vi "Autonomous Independent.vi"   [LabVIEW 2019]
doc: "This VI is called when autonomous begins, and will automatically be terminated when autonomous ends. You can carry out timed or sensor driven robot movement independently without needing to return to the caller."
uses:
  <vilib>/Rock Robotics/WPI/Utilities/WPI_GetSetVariantRefNum.vi
  <vilib>/Rock Robotics/Network Tables/NT Read String.vi
  <vilib>/Rock Robotics/Network Tables/NT Write Numeric Array.vi
  Robot Global Data.vi
panel:
  # "Be sure to right-click and choose Data Operations>>Make Current Value default if you want to save the array values with the VI"
types:
  T1 = typedef "WPI_JoystickDevRef.ctl" = cluster{"Device":T2}
  T2 = typedef "WPI_JoystickDeviceEnum.ctl" = enum16{"USB 0", "USB 1", "USB 2", "USB 3", "USB 4", "USB 5"}
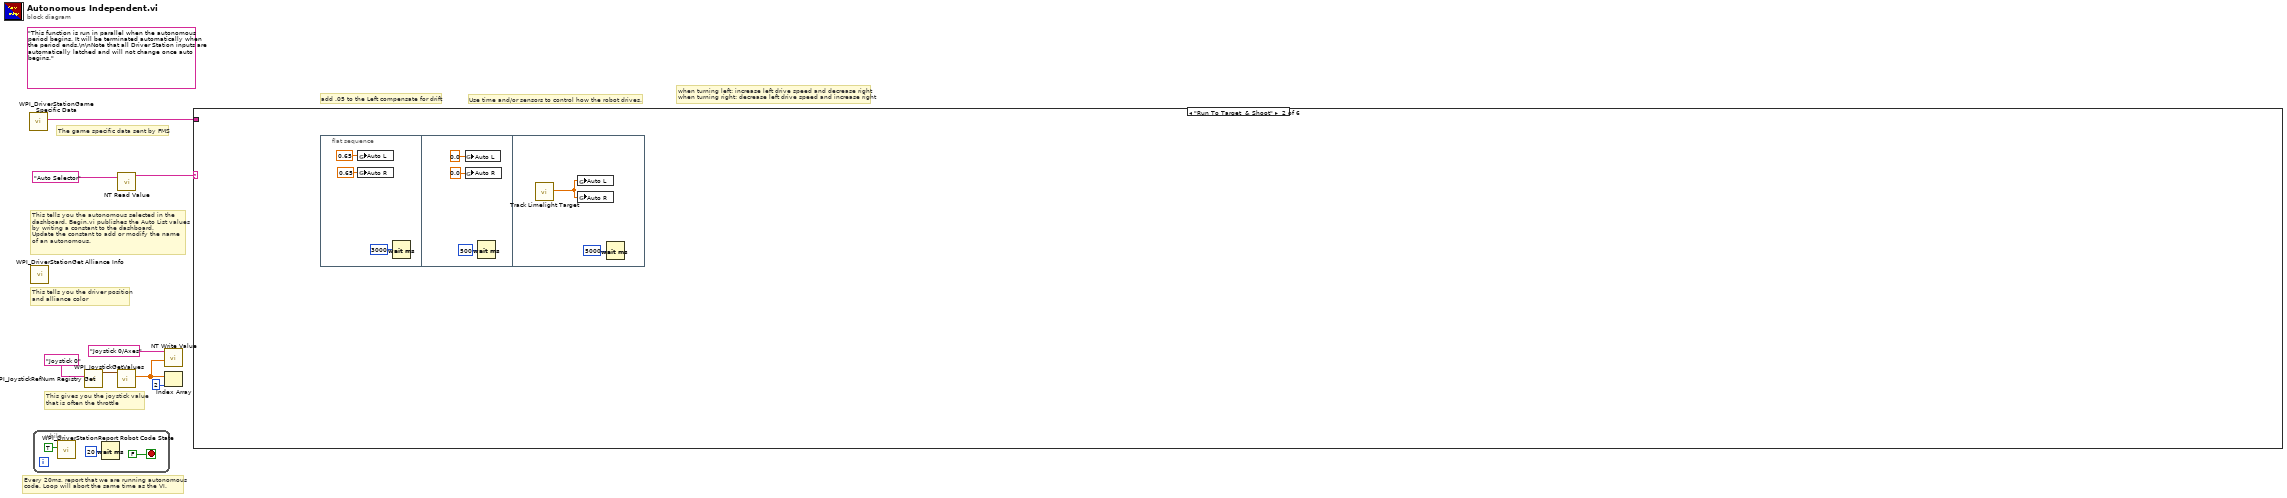
[diagram p0: block diagram]
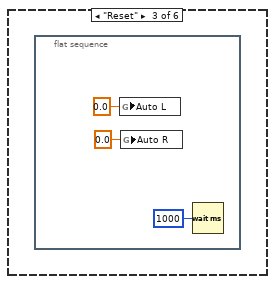
[diagram p3: hidden frame]
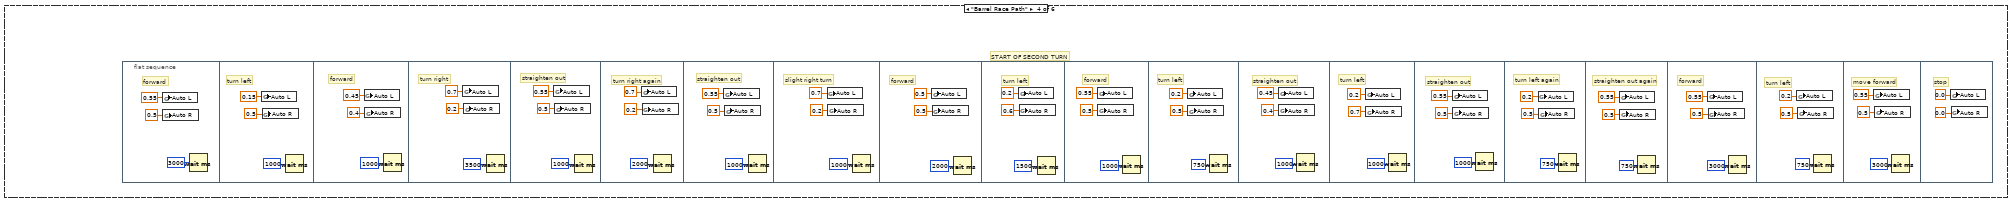
[diagram p4: hidden frame]
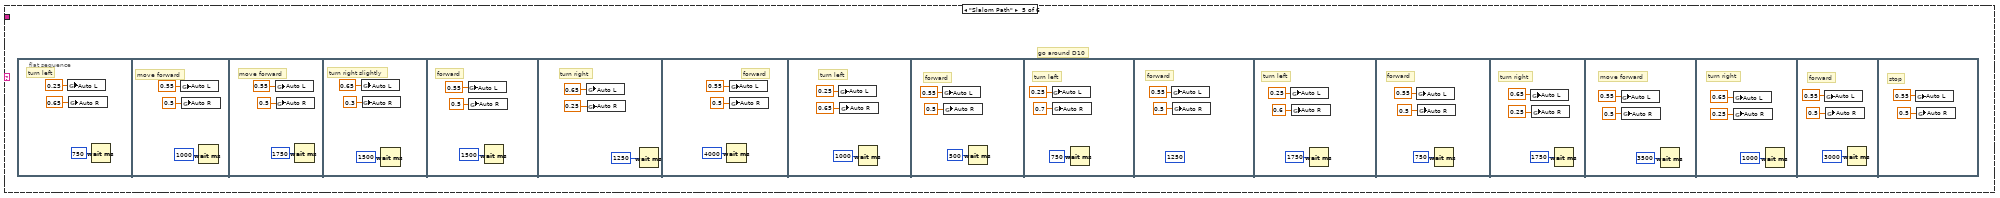
[diagram p5: hidden frame]
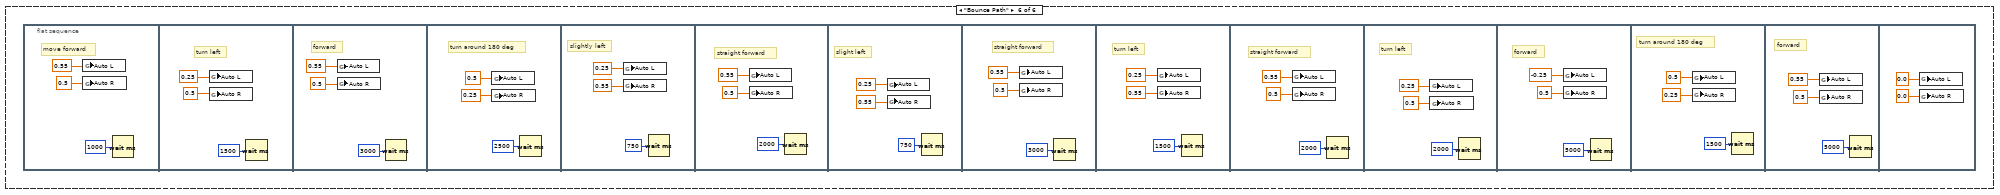
[diagram p6: hidden frame]
diagram:
  (unwired) "This function is run in parallel when the autonomous period begins. It will be terminated automatically when the period ends.\n\nNote that all Driver Station inputs are automatically latched and will not change once auto begins."
  # "add .05 to the Left compensate for drift"
  # "when turning left: increase left drive speed and decrease right\nwhen turning right: decrease left drive speed and increase right"
  # "The game specific data sent by FMS"
  # "This tells you the autonomous selected in the \ndashboard. Begin.vi publishes the Auto List values\nby writing a constant to the dashboard.\nUpdate the constant to add or modify the name\nof an autonomous."
  # "Every 20ms, report that we are running autonomous\ncode. Loop will abort the same time as the VI."
  # "This gives you the joystick value\nthat is often the throttle"
  # "Use time and/or sensors to control how the robot drives."
  # "This tells you the driver position\nand alliance color"
  n1 = call <vilib>:"WPI_DriverStationGame Specific Data.vi"() -> ("Game Specific Data"=w1:string)  [unwired: 11 in]
  n2 = call <vilib>:"WPI_DriverStationGet Alliance Info.vi"() -> ()  [unwired: 12 out]
  n3 = while {
    stop <- FALSE stop-if-true
    n4 = call <vilib>:"WPI_DriverStationReport Robot Code State.vi"("Autonomous"=TRUE) -> ()  [unwired: 10 in, 1 out]
    n5 = Wait (ms)(milliseconds to wait=u32 20) -> ()  [unwired: 1 out]
  }
  n6 = call <vilib>:"WPI_JoystickRefNum Registry Get.vi"("refnum name"="Joystick 0") -> ("JoystickDevRef"=w7:T1)  [unwired: 1 in, 9 out]
  n7 = call <vilib>:"WPI_JoystickGetValues.vi"("JoystickDevRef"=w7) -> ("Axes"=w3:dbl[])  [unwired: 6 in, 4 out]
  n8 = call-poly <vilib>:"NT Read Value.vi"("Name"="Auto Selector") -> ("String"=w4:string)  [unwired: 9 in, 1 out]
  n9 = call-poly <vilib>:"NT Write Value.vi"("Numeric Array"=w3, "Name"="Joystick 0/Axes") -> ()  [unwired: 9 in, 1 out]
  n10 = Index Array(array=w3, index=2) -> ()  [unwired: 1 out]
  n11 = case shown="\"Run To Target  & Shoot\"" w4 {
    tunnel: w1 -> [_ _ _ _ _ _]
    frame Default {
      # "You can put your main auto here, or you can right-click on the case and make any\nother frame be the default case."
      # "This is the frame that will execute if no selection is made, or if it is not recognized"
    }
    frame "Run To Target  & Shoot" {
      n12 = flat-sequence {
        frame #0 {
          n13 = global write "Robot Global Data.vi" "Auto L"(0.65 ("Auto L")) -> ()
          n14 = global write "Robot Global Data.vi" "Auto R"(0.65 ("Auto R")) -> ()
          n15 = Wait (ms)(milliseconds to wait=u32 3000) -> ()  [unwired: 1 out]
        }
        frame #1 {
          n16 = global write "Robot Global Data.vi" "Auto L"(0.0 ("Auto L")) -> ()
          n17 = global write "Robot Global Data.vi" "Auto R"(0.0 ("Auto R")) -> ()
          n18 = Wait (ms)(milliseconds to wait=u32 500) -> ()  [unwired: 1 out]
        }
        frame #2 {
          n19 = call "Track Limelight Target.vi"() -> ("Joystick X"=w19:dbl)  [unwired: 11 in]
          n20 = global write "Robot Global Data.vi" "Auto L"(w19) -> ()
          n21 = global write "Robot Global Data.vi" "Auto R"(w19) -> ()
          n22 = Wait (ms)(milliseconds to wait=u32 5000) -> ()  [unwired: 1 out]
        }
      }
    }
    frame "Reset" {
      n23 = flat-sequence {
        frame #0 {
          n24 = global write "Robot Global Data.vi" "Auto L"(0.0 ("Auto L")) -> ()
          n25 = global write "Robot Global Data.vi" "Auto R"(0.0 ("Auto R")) -> ()
          n26 = Wait (ms)(milliseconds to wait=u32 1000) -> ()  [unwired: 1 out]
        }
      }
    }
    frame "Barrel Race Path" {
      # "START OF SECOND TURN"
      n27 = flat-sequence {
        frame #0 {
          # "forward"
          n28 = global write "Robot Global Data.vi" "Auto L"(0.55 ("Auto X")) -> ()
          n29 = global write "Robot Global Data.vi" "Auto R"(0.5 ("Auto Y")) -> ()
          n30 = Wait (ms)(milliseconds to wait=u32 3000) -> ()  [unwired: 1 out]
        }
        frame #1 {
          # "turn left"
          n31 = global write "Robot Global Data.vi" "Auto L"(0.15 ("Auto X")) -> ()
          n32 = global write "Robot Global Data.vi" "Auto R"(0.5 ("Auto Y")) -> ()
          n33 = Wait (ms)(milliseconds to wait=u32 1000) -> ()  [unwired: 1 out]
        }
        frame #2 {
          # "forward"
          n34 = global write "Robot Global Data.vi" "Auto L"(0.45 ("Auto X")) -> ()
          n35 = global write "Robot Global Data.vi" "Auto R"(0.4 ("Auto Y")) -> ()
          n36 = Wait (ms)(milliseconds to wait=u32 1000) -> ()  [unwired: 1 out]
        }
        frame #3 {
          # "turn right"
          n37 = global write "Robot Global Data.vi" "Auto L"(0.7 ("Auto X")) -> ()
          n38 = global write "Robot Global Data.vi" "Auto R"(0.2 ("Auto Y")) -> ()
          n39 = Wait (ms)(milliseconds to wait=u32 3500) -> ()  [unwired: 1 out]
        }
        frame #4 {
          # "straighten out"
          n40 = global write "Robot Global Data.vi" "Auto L"(0.55 ("Auto X")) -> ()
          n41 = global write "Robot Global Data.vi" "Auto R"(0.5 ("Auto Y")) -> ()
          n42 = Wait (ms)(milliseconds to wait=u32 1000) -> ()  [unwired: 1 out]
        }
        frame #5 {
          # "turn right again"
          n43 = global write "Robot Global Data.vi" "Auto L"(0.7 ("Auto X")) -> ()
          n44 = global write "Robot Global Data.vi" "Auto R"(0.2 ("Auto Y")) -> ()
          n45 = Wait (ms)(milliseconds to wait=u32 2000) -> ()  [unwired: 1 out]
        }
        frame #6 {
          # "straighten out"
          n46 = global write "Robot Global Data.vi" "Auto L"(0.55 ("Auto X")) -> ()
          n47 = global write "Robot Global Data.vi" "Auto R"(0.5 ("Auto Y")) -> ()
          n48 = Wait (ms)(milliseconds to wait=u32 1000) -> ()  [unwired: 1 out]
        }
        frame #7 {
          # "slight right turn"
          n49 = global write "Robot Global Data.vi" "Auto L"(0.7 ("Auto X")) -> ()
          n50 = global write "Robot Global Data.vi" "Auto R"(0.2 ("Auto Y")) -> ()
          n51 = Wait (ms)(milliseconds to wait=u32 1000) -> ()  [unwired: 1 out]
        }
        frame #8 {
          # "forward"
          n52 = global write "Robot Global Data.vi" "Auto L"(0.5 ("Auto X")) -> ()
          n53 = global write "Robot Global Data.vi" "Auto R"(0.5 ("Auto Y")) -> ()
          n54 = Wait (ms)(milliseconds to wait=u32 2000) -> ()  [unwired: 1 out]
        }
        frame #9 {
          # "turn left"
          n55 = global write "Robot Global Data.vi" "Auto L"(0.2 ("Auto X")) -> ()
          n56 = global write "Robot Global Data.vi" "Auto R"(0.6 ("Auto Y")) -> ()
          n57 = Wait (ms)(milliseconds to wait=u32 1500) -> ()  [unwired: 1 out]
        }
        frame #10 {
          # "forward"
          n58 = global write "Robot Global Data.vi" "Auto L"(0.55 ("Auto X")) -> ()
          n59 = global write "Robot Global Data.vi" "Auto R"(0.5 ("Auto Y")) -> ()
          n60 = Wait (ms)(milliseconds to wait=u32 1000) -> ()  [unwired: 1 out]
        }
        frame #11 {
          # "turn left"
          n61 = global write "Robot Global Data.vi" "Auto L"(0.2 ("Auto X")) -> ()
          n62 = global write "Robot Global Data.vi" "Auto R"(0.5 ("Auto Y")) -> ()
          n63 = Wait (ms)(milliseconds to wait=u32 750) -> ()  [unwired: 1 out]
        }
        frame #12 {
          # "straighten out"
          n64 = global write "Robot Global Data.vi" "Auto L"(0.45 ("Auto X")) -> ()
          n65 = global write "Robot Global Data.vi" "Auto R"(0.4 ("Auto Y")) -> ()
          n66 = Wait (ms)(milliseconds to wait=u32 1000) -> ()  [unwired: 1 out]
        }
        frame #13 {
          # "turn left"
          n67 = global write "Robot Global Data.vi" "Auto L"(0.2 ("Auto X")) -> ()
          n68 = global write "Robot Global Data.vi" "Auto R"(0.7 ("Auto Y")) -> ()
          n69 = Wait (ms)(milliseconds to wait=u32 1000) -> ()  [unwired: 1 out]
        }
        frame #14 {
          # "straighten out"
          n70 = global write "Robot Global Data.vi" "Auto L"(0.55 ("Auto X")) -> ()
          n71 = global write "Robot Global Data.vi" "Auto R"(0.5 ("Auto Y")) -> ()
          n72 = Wait (ms)(milliseconds to wait=u32 1000) -> ()  [unwired: 1 out]
        }
        frame #15 {
          # "turn left again"
          n73 = global write "Robot Global Data.vi" "Auto L"(0.2 ("Auto X")) -> ()
          n74 = global write "Robot Global Data.vi" "Auto R"(0.5 ("Auto Y")) -> ()
          n75 = Wait (ms)(milliseconds to wait=u32 750) -> ()  [unwired: 1 out]
        }
        frame #16 {
          # "straighten out again"
          n76 = global write "Robot Global Data.vi" "Auto L"(0.55 ("Auto X")) -> ()
          n77 = global write "Robot Global Data.vi" "Auto R"(0.5 ("Auto Y")) -> ()
          n78 = Wait (ms)(milliseconds to wait=u32 750) -> ()  [unwired: 1 out]
        }
        frame #17 {
          # "forward"
          n79 = global write "Robot Global Data.vi" "Auto L"(0.55 ("Auto X")) -> ()
          n80 = global write "Robot Global Data.vi" "Auto R"(0.5 ("Auto Y")) -> ()
          n81 = Wait (ms)(milliseconds to wait=u32 3000) -> ()  [unwired: 1 out]
        }
        frame #18 {
          # "turn left"
          n82 = global write "Robot Global Data.vi" "Auto L"(0.2 ("Auto X")) -> ()
          n83 = global write "Robot Global Data.vi" "Auto R"(0.5 ("Auto Y")) -> ()
          n84 = Wait (ms)(milliseconds to wait=u32 750) -> ()  [unwired: 1 out]
        }
        frame #19 {
          # "move forward"
          n85 = global write "Robot Global Data.vi" "Auto L"(0.55 ("Auto X")) -> ()
          n86 = global write "Robot Global Data.vi" "Auto R"(0.5 ("Auto Y")) -> ()
          n87 = Wait (ms)(milliseconds to wait=u32 3000) -> ()  [unwired: 1 out]
        }
        frame #20 {
          # "stop"
          n88 = global write "Robot Global Data.vi" "Auto L"(0.0 ("Auto X")) -> ()
          n89 = global write "Robot Global Data.vi" "Auto R"(0.0 ("Auto Y")) -> ()
        }
      }
    }
    frame "Slalom Path" {
      # "go around D10"
      n90 = flat-sequence {
        frame #0 {
          # "turn left"
          n91 = global write "Robot Global Data.vi" "Auto L"(0.25 ("Auto L")) -> ()
          n92 = global write "Robot Global Data.vi" "Auto R"(0.65 ("Auto R")) -> ()
          n93 = Wait (ms)(milliseconds to wait=u32 750) -> ()  [unwired: 1 out]
        }
        frame #1 {
          # "move forward"
          n94 = global write "Robot Global Data.vi" "Auto L"(0.55 ("Auto L")) -> ()
          n95 = global write "Robot Global Data.vi" "Auto R"(0.5 ("Auto R")) -> ()
          n96 = Wait (ms)(milliseconds to wait=u32 1000) -> ()  [unwired: 1 out]
        }
        frame #2 {
          # "move forward"
          n97 = global write "Robot Global Data.vi" "Auto L"(0.55 ("Auto L")) -> ()
          n98 = global write "Robot Global Data.vi" "Auto R"(0.5 ("Auto R")) -> ()
          n99 = Wait (ms)(milliseconds to wait=u32 1750) -> ()  [unwired: 1 out]
        }
        frame #3 {
          # "turn right slightly"
          n100 = global write "Robot Global Data.vi" "Auto L"(0.65 ("Auto L")) -> ()
          n101 = global write "Robot Global Data.vi" "Auto R"(0.3 ("Auto R")) -> ()
          n102 = Wait (ms)(milliseconds to wait=u32 1500) -> ()  [unwired: 1 out]
        }
        frame #4 {
          # "forward"
          n103 = global write "Robot Global Data.vi" "Auto L"(0.55 ("Auto L")) -> ()
          n104 = global write "Robot Global Data.vi" "Auto R"(0.5 ("Auto R")) -> ()
          n105 = Wait (ms)(milliseconds to wait=u32 1500) -> ()  [unwired: 1 out]
        }
        frame #5 {
          # "turn right"
          n106 = global write "Robot Global Data.vi" "Auto L"(0.65 ("Auto L")) -> ()
          n107 = global write "Robot Global Data.vi" "Auto R"(0.25 ("Auto R")) -> ()
          n108 = Wait (ms)(milliseconds to wait=u32 1250) -> ()  [unwired: 1 out]
        }
        frame #6 {
          # "forward"
          n109 = Wait (ms)(milliseconds to wait=u32 4000) -> ()  [unwired: 1 out]
          n110 = global write "Robot Global Data.vi" "Auto L"(0.55 ("Auto L")) -> ()
          n111 = global write "Robot Global Data.vi" "Auto R"(0.5 ("Auto R")) -> ()
        }
        frame #7 {
          # "turn left"
          n112 = global write "Robot Global Data.vi" "Auto L"(0.25 ("Auto L")) -> ()
          n113 = global write "Robot Global Data.vi" "Auto R"(0.65 ("Auto R")) -> ()
          n114 = Wait (ms)(milliseconds to wait=u32 1000) -> ()  [unwired: 1 out]
        }
        frame #8 {
          # "forward"
          n115 = global write "Robot Global Data.vi" "Auto L"(0.55 ("Auto L")) -> ()
          n116 = global write "Robot Global Data.vi" "Auto R"(0.5 ("Auto R")) -> ()
          n117 = Wait (ms)(milliseconds to wait=u32 500) -> ()  [unwired: 1 out]
        }
        frame #9 {
          # "turn left"
          n118 = global write "Robot Global Data.vi" "Auto L"(0.25 ("Auto L")) -> ()
          n119 = global write "Robot Global Data.vi" "Auto R"(0.7 ("Auto R")) -> ()
          n120 = Wait (ms)(milliseconds to wait=u32 750) -> ()  [unwired: 1 out]
        }
        frame #10 {
          (unwired) u32 1250 ("milliseconds to wait")
          # "forward"
          n121 = global write "Robot Global Data.vi" "Auto L"(0.55 ("Auto L")) -> ()
          n122 = global write "Robot Global Data.vi" "Auto R"(0.5 ("Auto R")) -> ()
        }
        frame #11 {
          # "turn left"
          n123 = global write "Robot Global Data.vi" "Auto L"(0.25 ("Auto L")) -> ()
          n124 = global write "Robot Global Data.vi" "Auto R"(0.6 ("Auto R")) -> ()
          n125 = Wait (ms)(milliseconds to wait=u32 1750) -> ()  [unwired: 1 out]
        }
        frame #12 {
          # "forward"
          n126 = global write "Robot Global Data.vi" "Auto L"(0.55 ("Auto L")) -> ()
          n127 = global write "Robot Global Data.vi" "Auto R"(0.5 ("Auto R")) -> ()
          n128 = Wait (ms)(milliseconds to wait=u32 750) -> ()  [unwired: 1 out]
        }
        frame #13 {
          # "turn right"
          n129 = global write "Robot Global Data.vi" "Auto L"(0.65 ("Auto L")) -> ()
          n130 = global write "Robot Global Data.vi" "Auto R"(0.25 ("Auto R")) -> ()
          n131 = Wait (ms)(milliseconds to wait=u32 1750) -> ()  [unwired: 1 out]
        }
        frame #14 {
          # "move forward"
          n132 = global write "Robot Global Data.vi" "Auto L"(0.55 ("Auto L")) -> ()
          n133 = global write "Robot Global Data.vi" "Auto R"(0.5 ("Auto R")) -> ()
          n134 = Wait (ms)(milliseconds to wait=u32 3500) -> ()  [unwired: 1 out]
        }
        frame #15 {
          # "turn right"
          n135 = global write "Robot Global Data.vi" "Auto L"(0.65 ("Auto L")) -> ()
          n136 = global write "Robot Global Data.vi" "Auto R"(0.25 ("Auto R")) -> ()
          n137 = Wait (ms)(milliseconds to wait=u32 1000) -> ()  [unwired: 1 out]
        }
        frame #16 {
          # "forward"
          n138 = global write "Robot Global Data.vi" "Auto L"(0.55 ("Auto L")) -> ()
          n139 = global write "Robot Global Data.vi" "Auto R"(0.5 ("Auto R")) -> ()
          n140 = Wait (ms)(milliseconds to wait=u32 3000) -> ()  [unwired: 1 out]
        }
        frame #17 {
          # "stop"
          n141 = global write "Robot Global Data.vi" "Auto L"(0.55 ("Auto L")) -> ()
          n142 = global write "Robot Global Data.vi" "Auto R"(0.5 ("Auto R")) -> ()
        }
      }
    }
    frame "Bounce Path" {
      n143 = flat-sequence {
        frame #0 {
          # "move forward"
          n144 = global write "Robot Global Data.vi" "Auto L"(0.55 ("Joystick X")) -> ()
          n145 = global write "Robot Global Data.vi" "Auto R"(0.5 ("Joystick Y")) -> ()
          n146 = Wait (ms)(milliseconds to wait=u32 1000) -> ()  [unwired: 1 out]
        }
        frame #1 {
          # "turn left"
          n147 = global write "Robot Global Data.vi" "Auto L"(0.25 ("Joystick X")) -> ()
          n148 = global write "Robot Global Data.vi" "Auto R"(0.5 ("Joystick Y")) -> ()
          n149 = Wait (ms)(milliseconds to wait=u32 1500) -> ()  [unwired: 1 out]
        }
        frame #2 {
          # "forward"
          n150 = global write "Robot Global Data.vi" "Auto L"(0.55 ("Joystick X")) -> ()
          n151 = global write "Robot Global Data.vi" "Auto R"(0.5 ("Joystick Y")) -> ()
          n152 = Wait (ms)(milliseconds to wait=u32 3000) -> ()  [unwired: 1 out]
        }
        frame #3 {
          # "turn around 180 deg"
          n153 = global write "Robot Global Data.vi" "Auto L"(0.5 ("Joystick X")) -> ()
          n154 = global write "Robot Global Data.vi" "Auto R"(0.25 ("Joystick Y")) -> ()
          n155 = Wait (ms)(milliseconds to wait=u32 2500) -> ()  [unwired: 1 out]
        }
        frame #4 {
          # "slightly left"
          n156 = global write "Robot Global Data.vi" "Auto L"(0.25 ("Joystick X")) -> ()
          n157 = global write "Robot Global Data.vi" "Auto R"(0.55 ("Joystick Y")) -> ()
          n158 = Wait (ms)(milliseconds to wait=u32 750) -> ()  [unwired: 1 out]
        }
        frame #5 {
          # "straight forward"
          n159 = global write "Robot Global Data.vi" "Auto L"(0.55 ("Joystick X")) -> ()
          n160 = global write "Robot Global Data.vi" "Auto R"(0.5 ("Joystick Y")) -> ()
          n161 = Wait (ms)(milliseconds to wait=u32 2000) -> ()  [unwired: 1 out]
        }
        frame #6 {
          # "slight left"
          n162 = global write "Robot Global Data.vi" "Auto L"(0.25 ("Joystick X")) -> ()
          n163 = global write "Robot Global Data.vi" "Auto R"(0.55 ("Joystick Y")) -> ()
          n164 = Wait (ms)(milliseconds to wait=u32 750) -> ()  [unwired: 1 out]
        }
        frame #7 {
          # "straight forward"
          n165 = global write "Robot Global Data.vi" "Auto L"(0.55 ("Joystick X")) -> ()
          n166 = global write "Robot Global Data.vi" "Auto R"(0.5 ("Joystick Y")) -> ()
          n167 = Wait (ms)(milliseconds to wait=u32 3000) -> ()  [unwired: 1 out]
        }
        frame #8 {
          # "turn left"
          n168 = global write "Robot Global Data.vi" "Auto L"(0.25 ("Joystick X")) -> ()
          n169 = global write "Robot Global Data.vi" "Auto R"(0.55 ("Joystick Y")) -> ()
          n170 = Wait (ms)(milliseconds to wait=u32 1500) -> ()  [unwired: 1 out]
        }
        frame #9 {
          # "straight forward"
          n171 = global write "Robot Global Data.vi" "Auto L"(0.55 ("Joystick X")) -> ()
          n172 = global write "Robot Global Data.vi" "Auto R"(0.5 ("Joystick Y")) -> ()
          n173 = Wait (ms)(milliseconds to wait=u32 2000) -> ()  [unwired: 1 out]
        }
        frame #10 {
          # "turn left"
          n174 = global write "Robot Global Data.vi" "Auto L"(0.25 ("Joystick X")) -> ()
          n175 = global write "Robot Global Data.vi" "Auto R"(0.5 ("Joystick Y")) -> ()
          n176 = Wait (ms)(milliseconds to wait=u32 2000) -> ()  [unwired: 1 out]
        }
        frame #11 {
          # "forward"
          n177 = global write "Robot Global Data.vi" "Auto L"(-0.25 ("Joystick X")) -> ()
          n178 = global write "Robot Global Data.vi" "Auto R"(0.5 ("Joystick Y")) -> ()
          n179 = Wait (ms)(milliseconds to wait=u32 5000) -> ()  [unwired: 1 out]
        }
        frame #12 {
          # "turn around 180 deg"
          n180 = global write "Robot Global Data.vi" "Auto L"(0.5 ("Joystick X")) -> ()
          n181 = global write "Robot Global Data.vi" "Auto R"(0.25 ("Joystick Y")) -> ()
          n182 = Wait (ms)(milliseconds to wait=u32 1500) -> ()  [unwired: 1 out]
        }
        frame #13 {
          # "forward"
          n183 = global write "Robot Global Data.vi" "Auto L"(0.55 ("Joystick X")) -> ()
          n184 = global write "Robot Global Data.vi" "Auto R"(0.5 ("Joystick Y")) -> ()
          n185 = Wait (ms)(milliseconds to wait=u32 5000) -> ()  [unwired: 1 out]
        }
        frame #14 {
          n186 = global write "Robot Global Data.vi" "Auto L"(0.0 ("Joystick X")) -> ()
          n187 = global write "Robot Global Data.vi" "Auto R"(0.0 ("Joystick Y")) -> ()
        }
      }
    }
  }
